vi "Create HTML.vi"(7 "FP Reference":refnum<class "Web Front Panel.lvclass">, 8 "error in (no error)":errorcluster, 10 "VI Identifier":string, 11 "Numeric In":refnum<class "Numeric.lvclass">) -> (0 "error out":errorcluster, 1 "js code for controls":string, 2 "js variables":string, 3 "Numeric Out":refnum<class "Numeric.lvclass">, 4 "script dependencies":string[](array[string]), 5 "HTML":string, 6 "js code for indicators":string)   [LabVIEW 2017, in "Front Panel Publisher.lvlib" / "Numeric.lvclass"]
uses:
  Numeric.lvclass
  Object_class/Object.lvclass
  Control_class/Control.lvclass
  Front Panel Publisher.lvlib
  Web Front Panel_class/Web Front Panel.lvclass
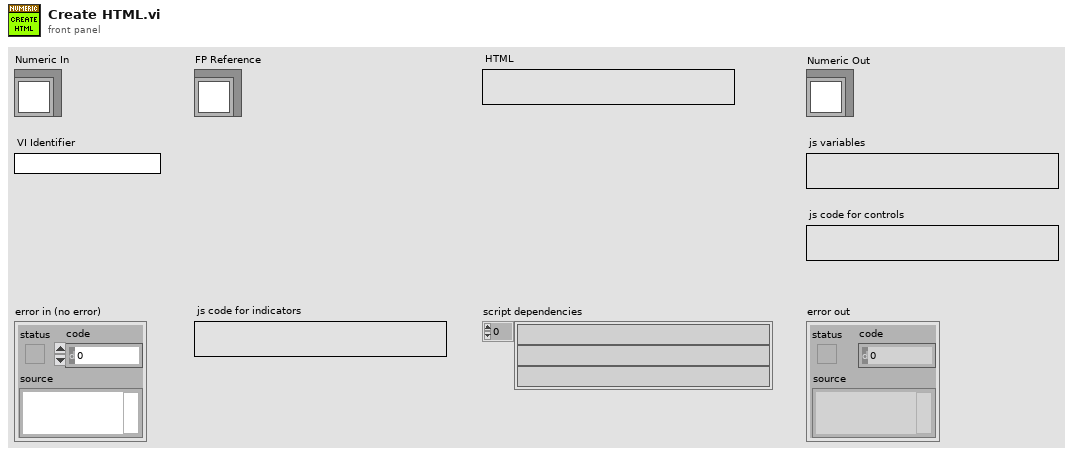
[diagram p1: front panel]
types:
  T1 = typedef "Front Panel Publisher.lvlib/Object.lvclass/Attributes.ctl" = cluster{"UID":i32, "Type":string, "Starting Location":T2, "Reference":refnum<vi>, "Cluster Component":bool, "Starting Rect Position":cluster{"Left":i16, "Top":i16}, "Owning Pane":refnum<vi>, "Master Total Rect Delta":T3}
  T2 = typedef "Front Panel Publisher.lvlib/Object.lvclass/Coordinates.ctl" = cluster{"Left":i32, "Top":i32, "Height":u32, "Width":u32}
  T3 = typedef "LVRectTypeDef.ctl" = cluster{"Left":i16, "Top":i16, "Right":i16, "Bottom":i16}
  T4 = typedef "Front Panel Publisher.lvlib/Control.lvclass/Attributes.ctl" = cluster{"Description":string, "Indicator":bool, "Default Value":variant, "Control Index":i32, "Label":refnum<class "Text.lvclass">, "Caption":refnum<class "Text.lvclass">, "Image b64":string, "No Control Index":bool, "Display Mode":T5}
  T5 = typedef "Front Panel Publisher.lvlib/Web Front Panel.lvclass/Enum - Control Display Mode.ctl" = enum16{"Value Only", "Value and Visibility", "Boolean Value Only", "Boolean Value and Visibility", "Control is Image", "Image and Visibility"}
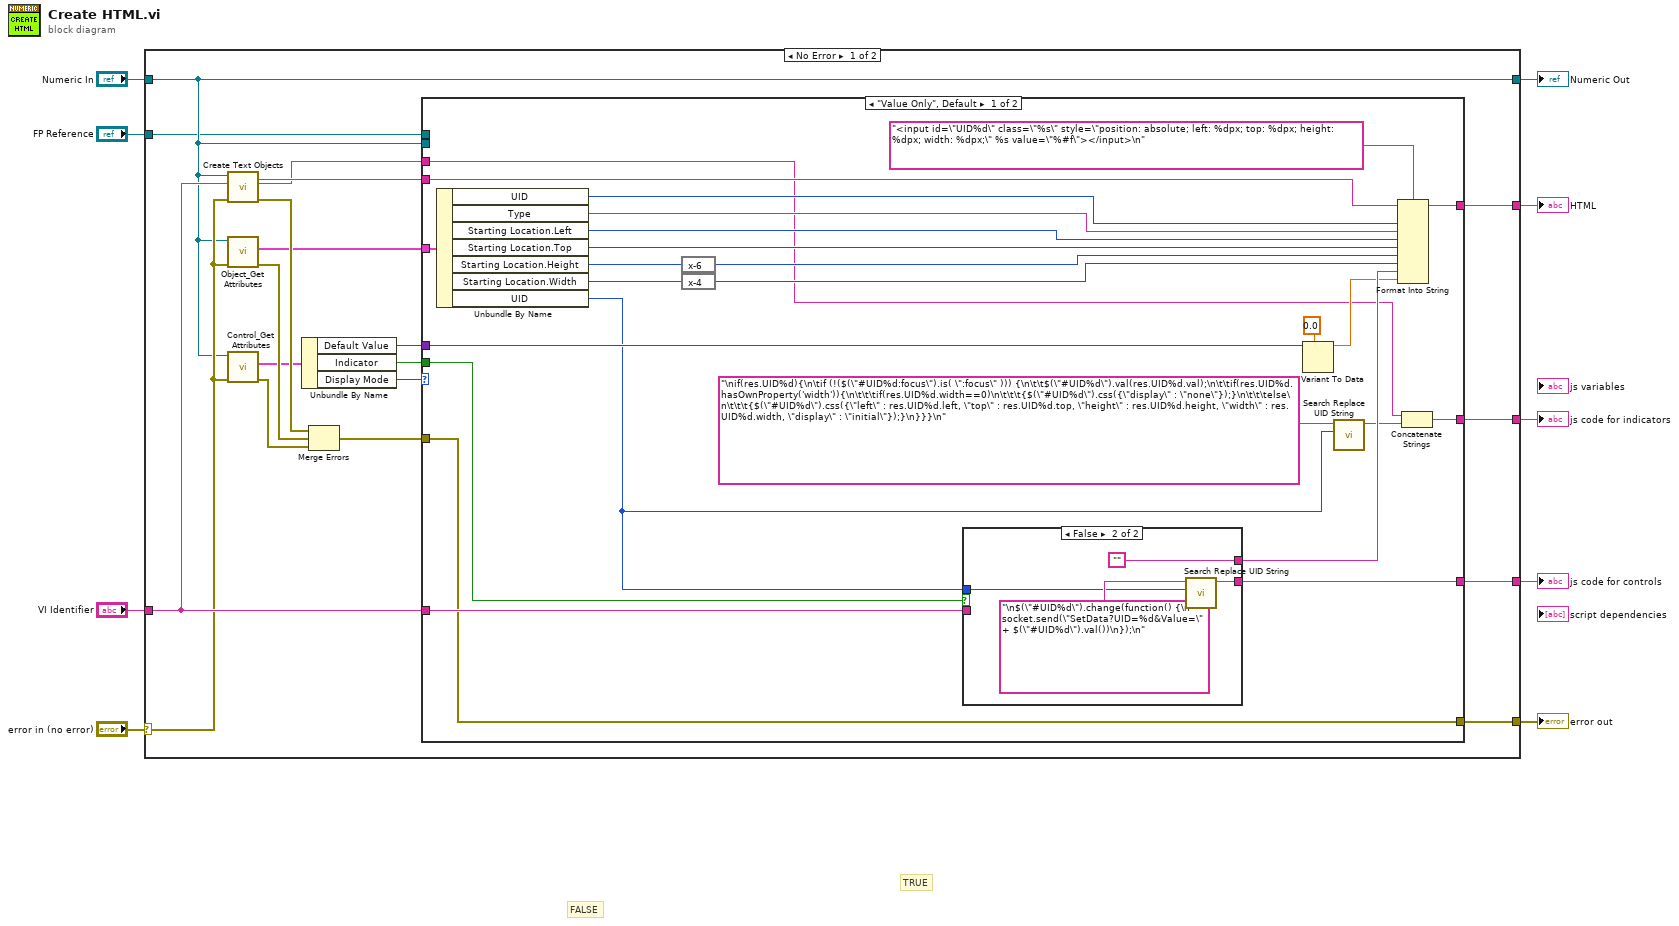
[diagram p0: block diagram]
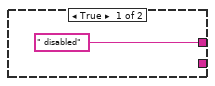
[diagram p2: hidden frame]
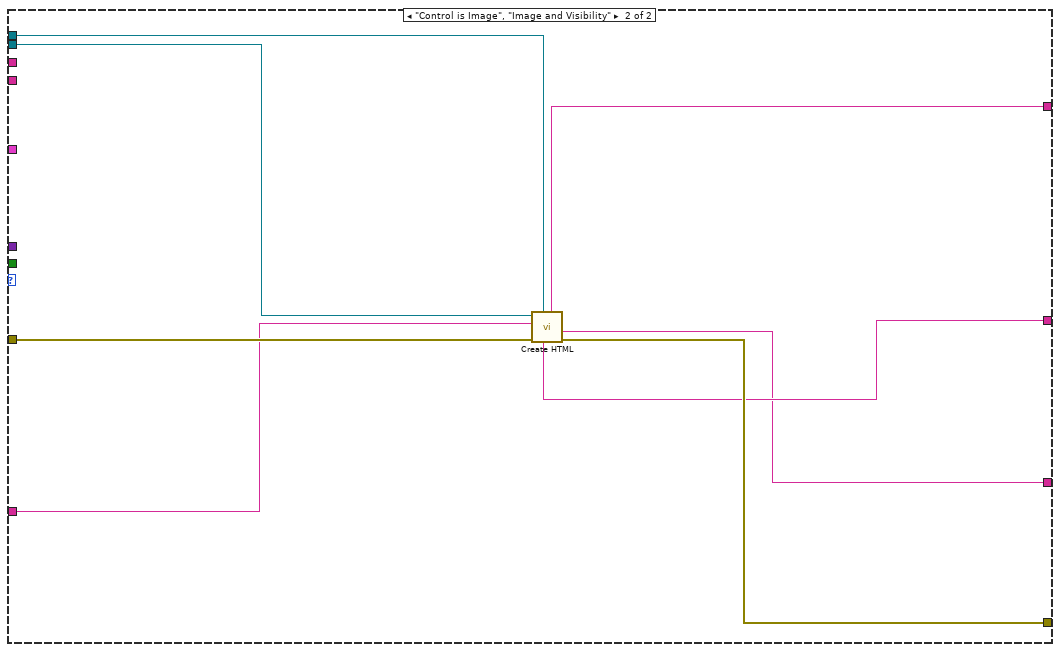
[diagram p3: hidden frame]
diagram:
  # "TRUE"
  # "FALSE"
  n1 = case shown="No Error" "error in (no error)" {
    selector: "error in (no error)" -> [w17 w68]
    tunnel: [w12 w68] -> w8
    tunnel: [w14 w67] -> w6
    tunnel: "Numeric In" -> [w14 w67]
    tunnel: [w25 _] -> w5
    tunnel: [w16 _] -> w4
    tunnel: [w21 _] -> w3
    tunnel: "VI Identifier" -> [w18 _]
    tunnel: "FP Reference" -> [w10 _]
    frame No Error {
      n2 = call-dynamic "Create Text Objects.vi"("error in (no error)"=w17, "VI Name"=w18, "Control In"=w14) -> ("error out"=w26:errorcluster, "JS Indicator"=w11:string, "HTML"=w19:string)  [unwired: 5 in, 1 out]
      n3 = call "Object_Get Attributes.vi"("error in (no error)"=w17, "Object In"=w14) -> ("error out"=w27:errorcluster, "Object Attributes"=w24:T1)  [unwired: 7 in, 1 out]
      n4 = call "Control_Get Attributes.vi"("error in (no error)"=w17, "Control In"=w14) -> ("error out"=w28:errorcluster, "Control Attributes"=w23:T4)  [unwired: 7 in, 1 out]
      n5 = Unbundle By Name(w23) -> ("Default Value"=w20:variant, "Indicator"=w22:bool, "Display Mode"=w15:T5)
      n6 = Merge Errors(w26, w27, w28) -> (w13:errorcluster)
      n7 = case shown="\"Value Only\", Default" w15 {
        tunnel: [w48 w62] -> w25
        tunnel: w24 -> [w47 _]
        tunnel: w22 -> [w42 _]
        tunnel: [w40 w60] -> w21
        tunnel: w20 -> [w38 _]
        tunnel: w19 -> [w36 _]
        tunnel: w18 -> [w35 w65]
        tunnel: [w31 w61] -> w16
        tunnel: w14 -> [_ w64]
        tunnel: w13 -> [w30 w66]
        tunnel: [w30 w63] -> w12
        tunnel: w11 -> [w29 _]
        tunnel: w10 -> [_ w59]
        frame "Value Only", Default {
          n8 = Unbundle By Name(w47) -> ("UID"=w52:i32, "Type"=w51:string, "Starting Location.Left"=w50:i32, "Starting Location.Top"=w49:i32, "Starting Location.Height"=w46:u32, "Starting Location.Width"=w44:u32, "UID"=w34:i32)
          n9 = expression code="x-6"(w46) -> (w45:u32)
          n10 = expression code="x-4"(w44) -> (w43:u32)
          n11 = case shown="False" w42 {
            tunnel: [" disabled" ""] -> w41
            tunnel: w34 -> [_ w55]
            tunnel: w35 -> [_ _]
            tunnel: [_ w56] -> w40
            frame True {
            }
            frame False {
              n12 = call "Search Replace UID String.vi"("UID"=w55, "Input String"="\n$(\"#UID%d\").change(function() {\n  socket.send(\"SetData?UID=%d&Value=\" + $(\"#UID%d\").val())\n});\n") -> ("Output String"=w56:string)  [unwired: 9 in]
            }
          }
          n13 = Variant To Data(type=0.0, Variant=w38) -> (data=w37:dbl)  [unwired: 1 in, 1 out]
          n14 = call "Search Replace UID String.vi"("UID"=w34, "Input String"="\nif(res.UID%d){\n\tif (!($(\"#UID%d:focus\").is( \":focus\" ))) {\n\t\t$(\"#UID%d\").val(res.UID%d.val);\n\t\tif(res.UID%d.hasOwnProperty('width')){\n\t\t\tif(res.UID%d.width==0)\n\t\t\t{$(\"#UID%d\").css({\"display\" : \"none\"});}\n\t\t\telse\n\t\t\t{$(\"#UID%d\").css({\"left\" : res.UID%d.left, \"top\" : res.UID%d.top, \"height\" : res.UID%d.height, \"width\" : res.UID%d.width, \"display\" : \"initial\"});}\n}}}\n") -> ("Output String"=w33:string)  [unwired: 9 in]
          n15 = Format Into String(format string="<input id=\"UID%d\" class=\"%s\" style=\"position: absolute; left: %dpx; top: %dpx; height: %dpx; width: %dpx;\" %s value=\"%#f\"></input>\n", initial string=w36, w52, w51, w50, w49, w45, w43, w41, w37) -> (resulting string=w48:string)  [unwired: 1 in, 1 out]
          n16 = Concatenate Strings(w29, w33) -> (w31:string)
        }
        frame "Control is Image", "Image and Visibility" {
          n17 = call-parent "Create HTML.vi"("FP Reference"=w59, "error in (no error)"=w66, "VI Identifier"=w65, "Control In"=w64) -> ("error out"=w63:errorcluster, "js code for controls"=w60:string, "HTML"=w62:string, "js code for indicators"=w61:string)  [unwired: 1 in, 3 out]
        }
      }
    }
    frame Error {
    }
  }
  "error out" <- w8
  "Numeric Out" <- w6
  "HTML" <- w5
  "js code for controls" <- w3
  "js code for indicators" <- w4
